vi "For Loop VI.vi"() -> ()   [LabVIEW 2020]
panel:
  in  "# of loops to iterate":dbl
  out "number (0 to 1)":dbl
  out "Loop iteration":i32
  # "For Loop"
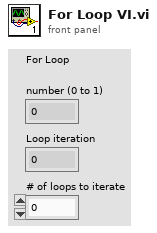
[diagram p1: front panel]
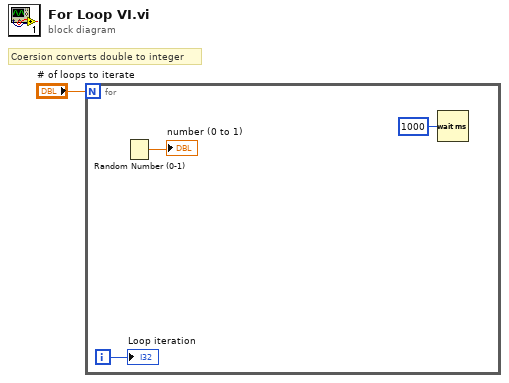
[diagram p0: block diagram]
diagram:
  # "Coersion converts double to integer"
  n1 = for {
    N: "# of loops to iterate" -> [_]
    i -> [w3]
    n2 = Random Number (0-1)() -> (number: 0 to 1=→"number (0 to 1)":dbl)
    n3 = Wait (ms)(milliseconds to wait=u32 1000) -> ()  [unwired: 1 out]
    "Loop iteration" <- w3
  }
